vi "write_csv.vi"   [LabVIEW 2024]
uses:
  <vilib>/Utility/file.llb/Write Delimited Spreadsheet (DBL).vi
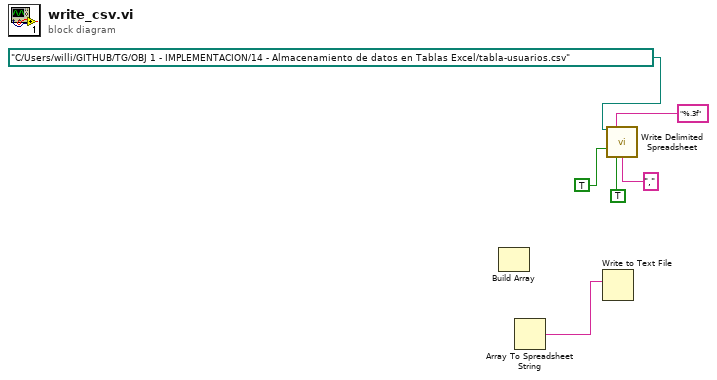
[diagram p0: block diagram]
diagram:
  n1 = Build Array() -> ()  [unwired: 3 in, 1 out]
  n2 = Array To Spreadsheet String() -> (spreadsheet string=w1:string)  [unwired: 3 in]
  n3 = Write to Text File(text=w1) -> ()  [unwired: 3 in, 3 out]
  n4 = call-poly <vilib>:"Write Delimited Spreadsheet.vi"("file path (dialog if empty)"=path "C:/Users/willi/GITHUB/TG/OBJ 1 - IMPLEMENTACION/14 - Almacenamiento de datos en Tablas Excel/tabla-usuarios.csv", "format (%.3f)"="%.3f", "append to file? (new file:F)"=TRUE, "transpose? (no:F)"=TRUE, "delimiter (\\t)"="," ("delimiter (\\t)")) -> ()  [unwired: 9 in, 2 out]
